vi "compare_command.vi"(11 "Command":string) -> (2 "Unknown":bool=TRUE, 3 "Count":i32=40)   [LabVIEW 2014]
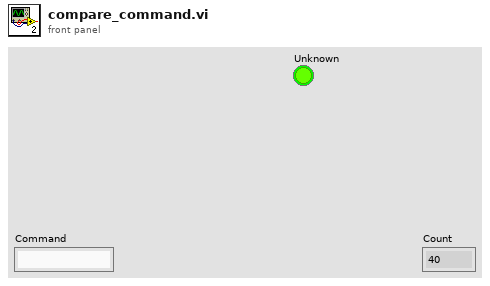
[diagram p1: front panel]
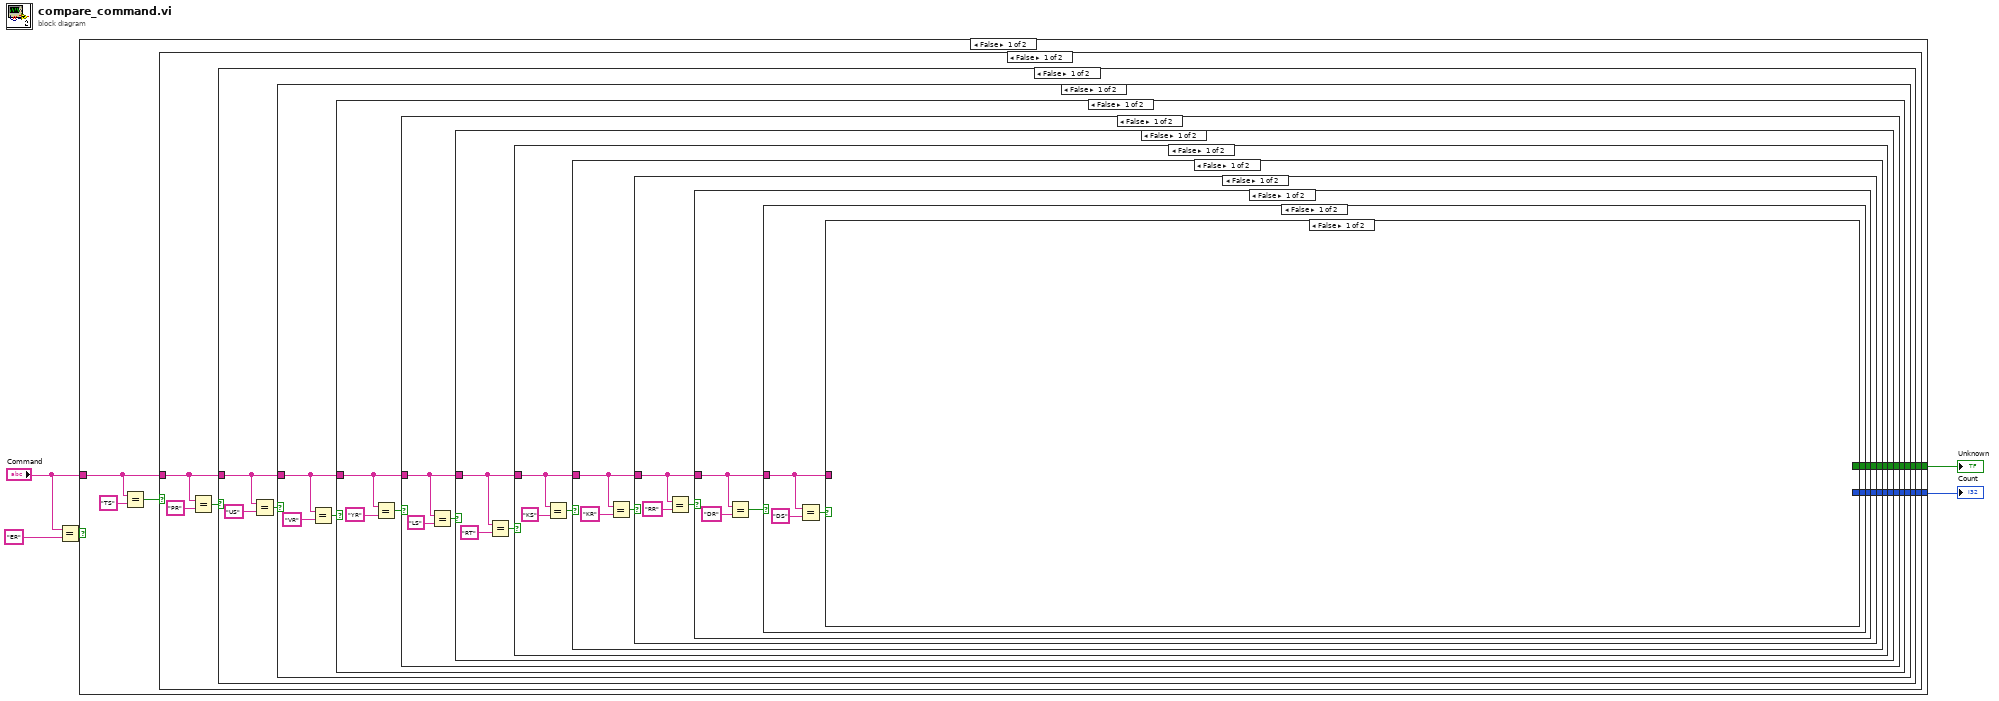
[diagram p0: block diagram]
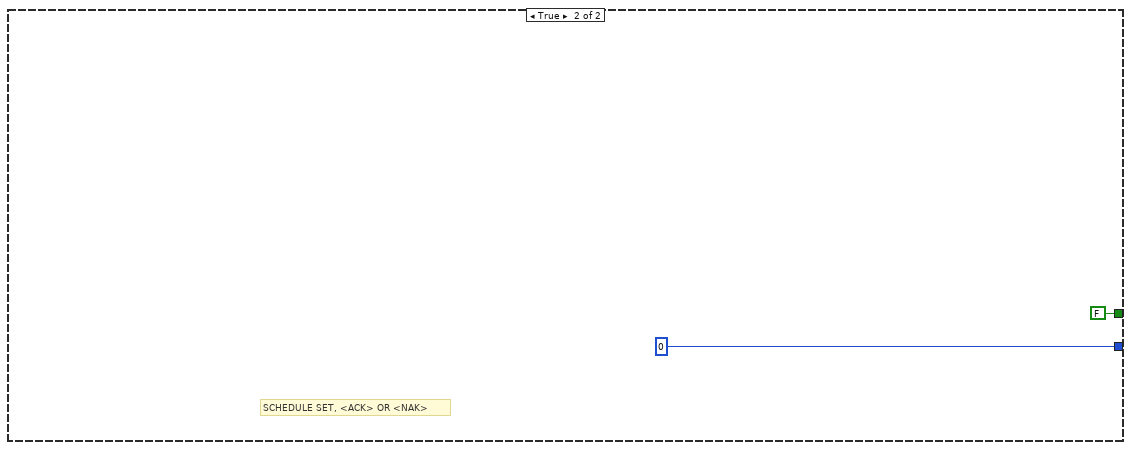
[diagram p2: hidden frame]
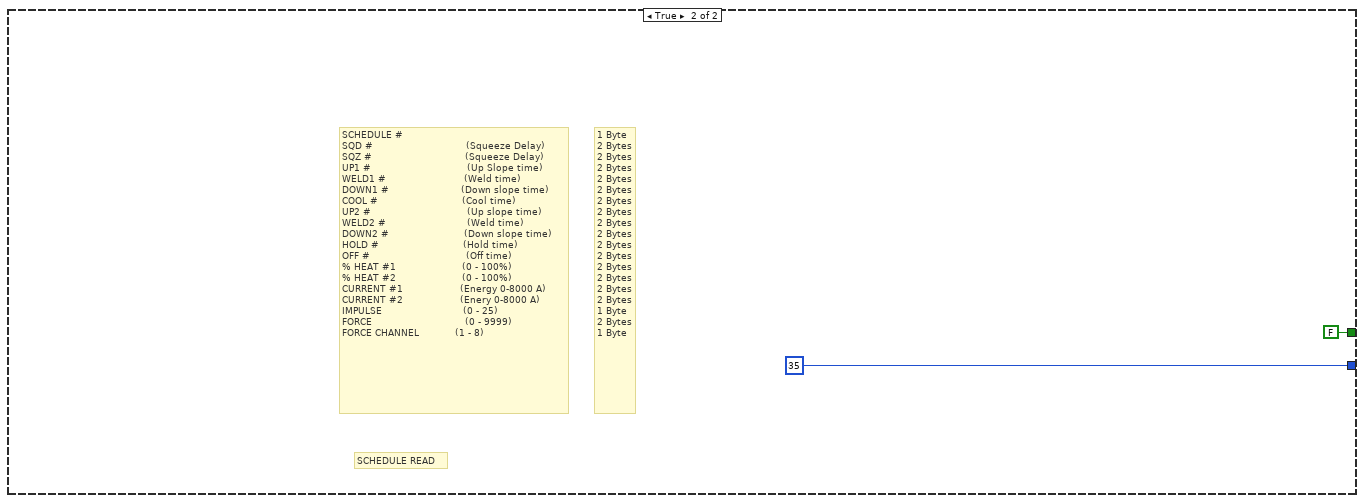
[diagram p3: hidden frame]
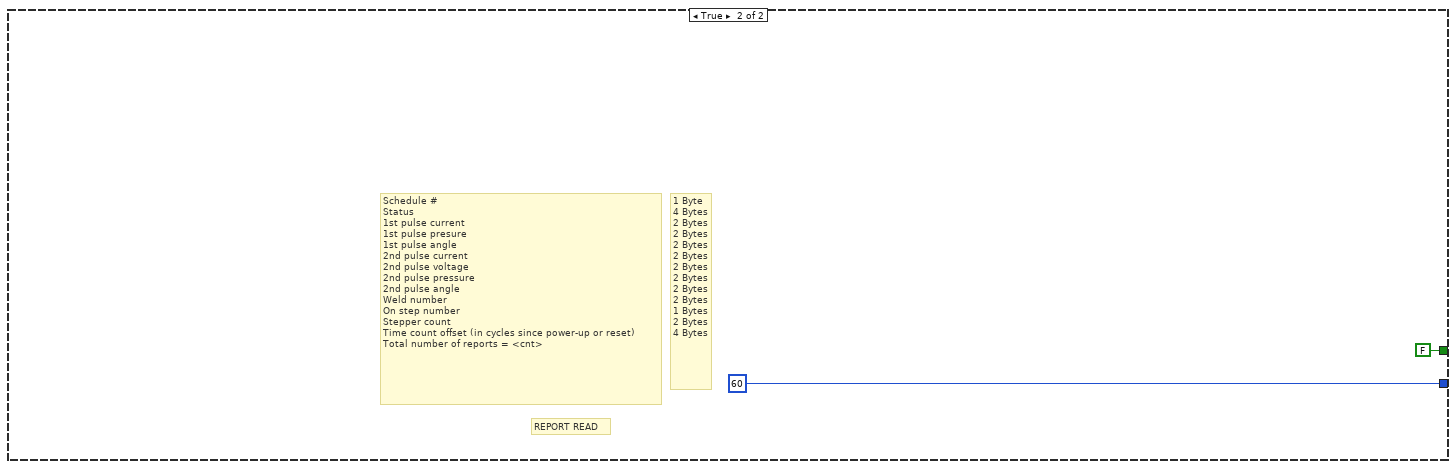
[diagram p4: hidden frame]
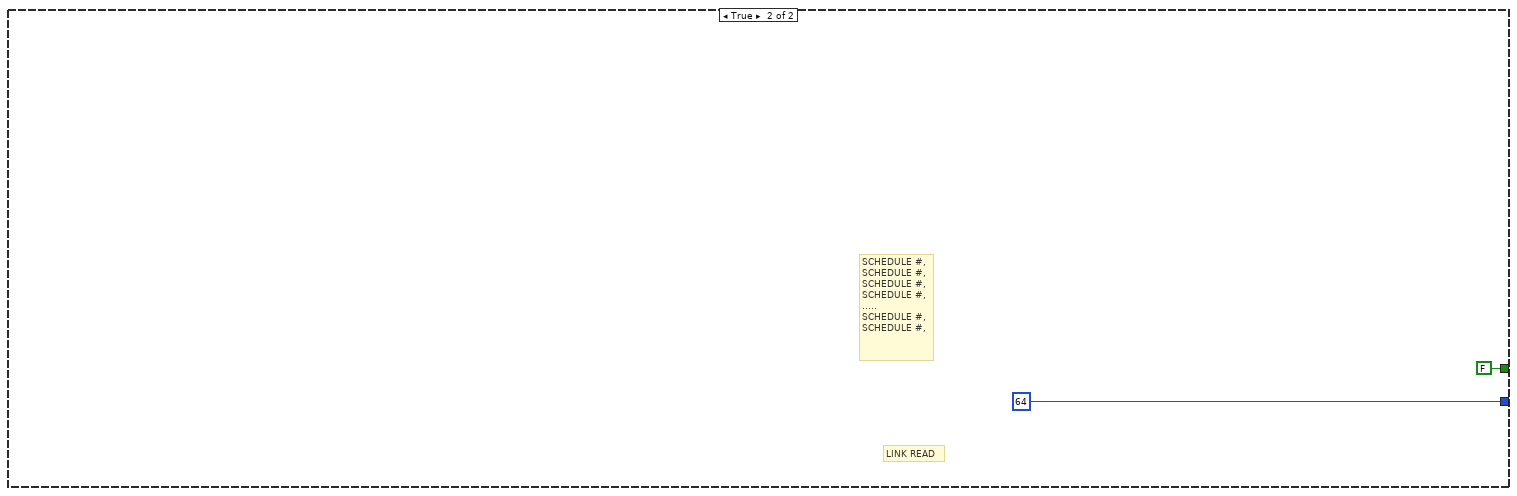
[diagram p5: hidden frame]
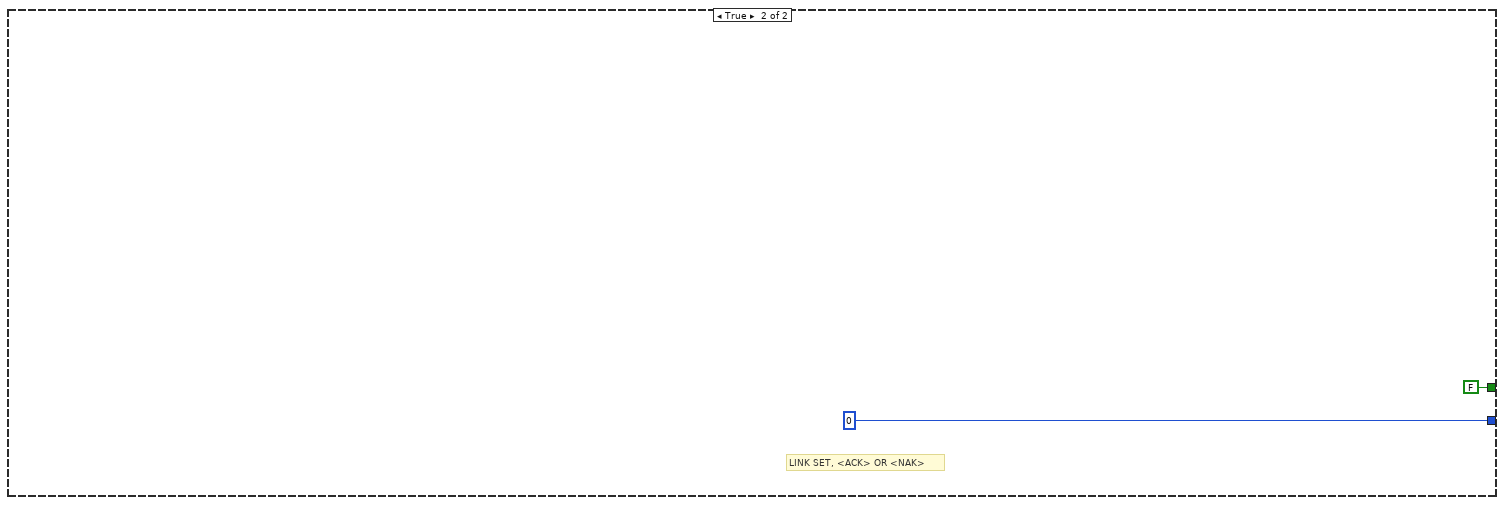
[diagram p6: hidden frame]
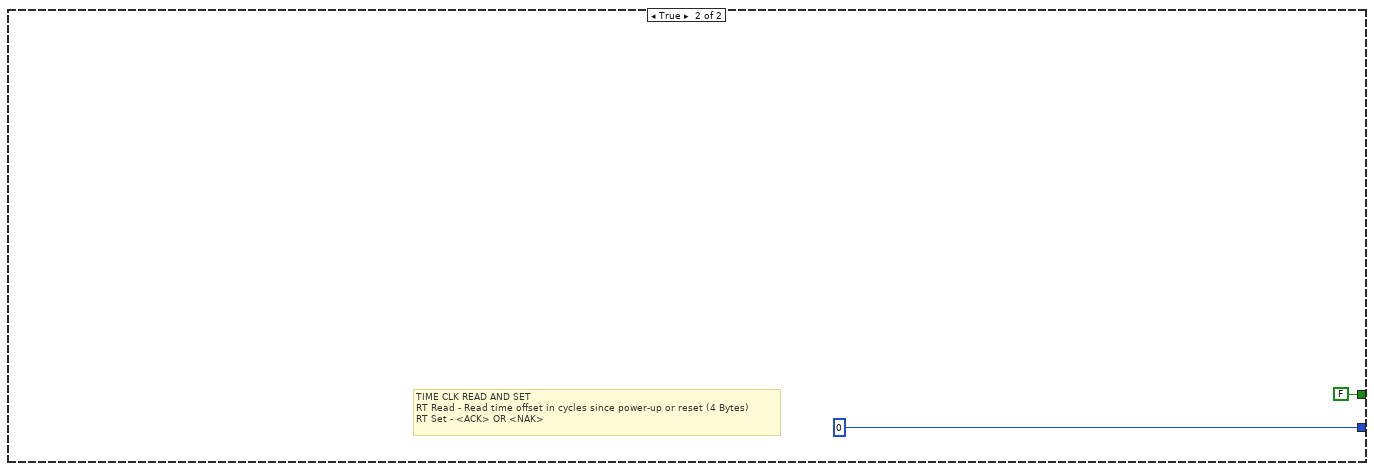
[diagram p7: hidden frame]
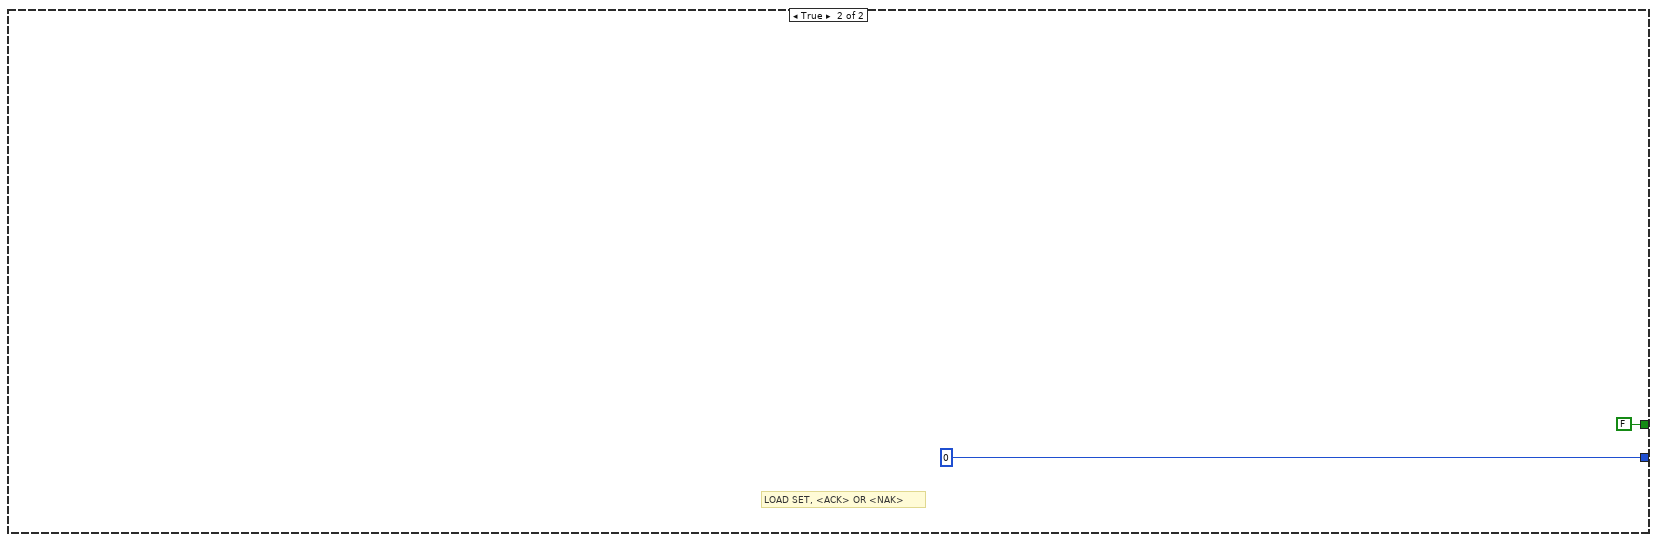
[diagram p8: hidden frame]
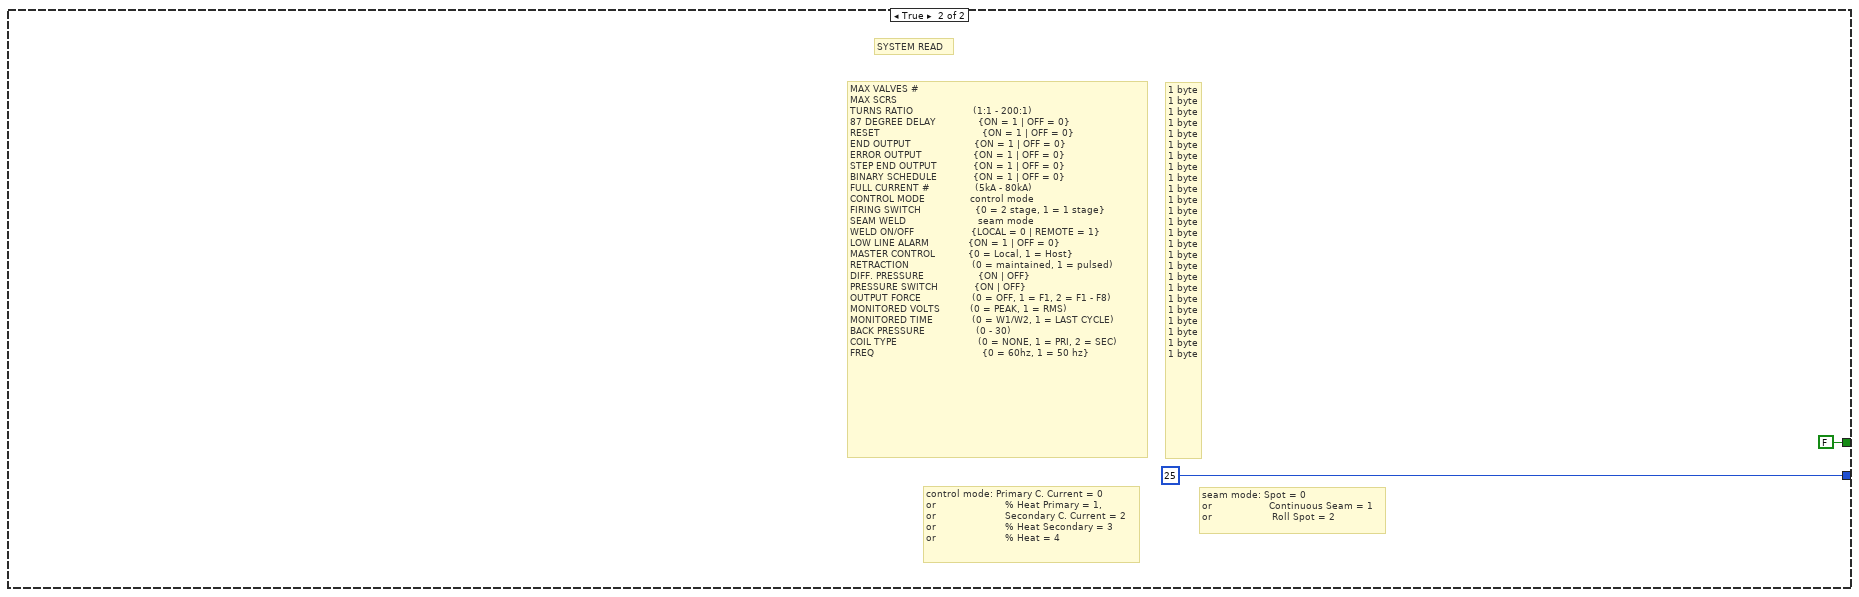
[diagram p9: hidden frame]
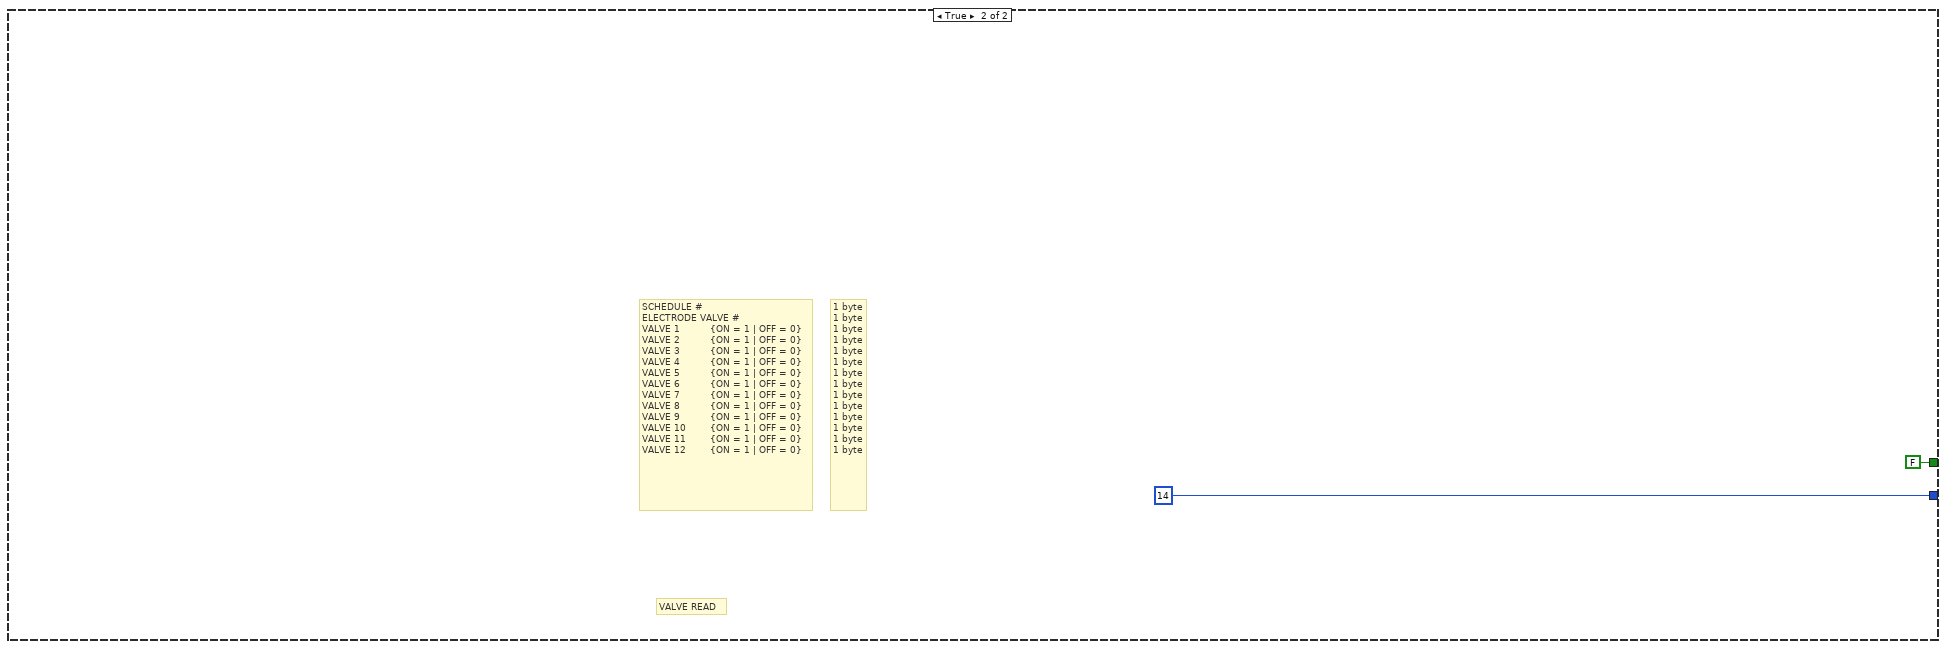
[diagram p10: hidden frame]
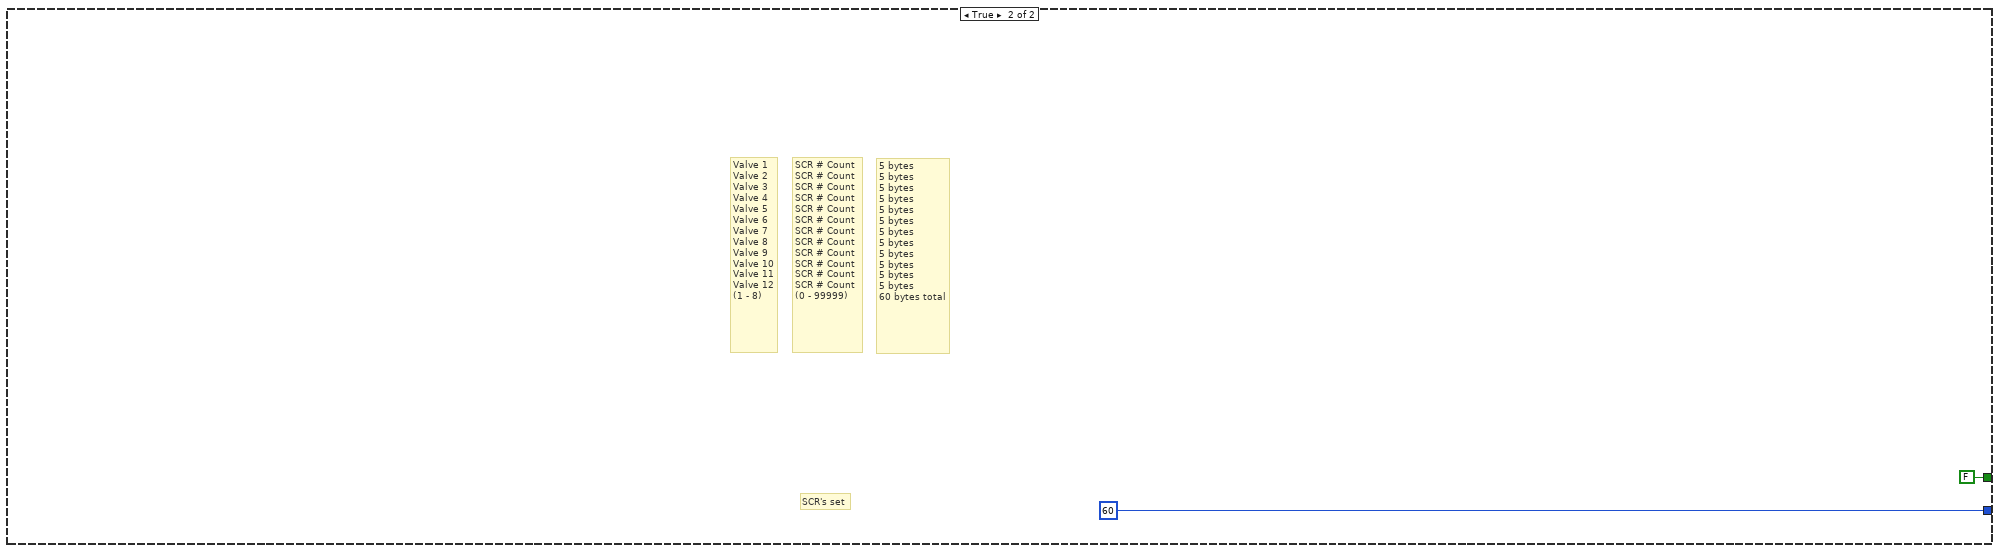
[diagram p11: hidden frame]
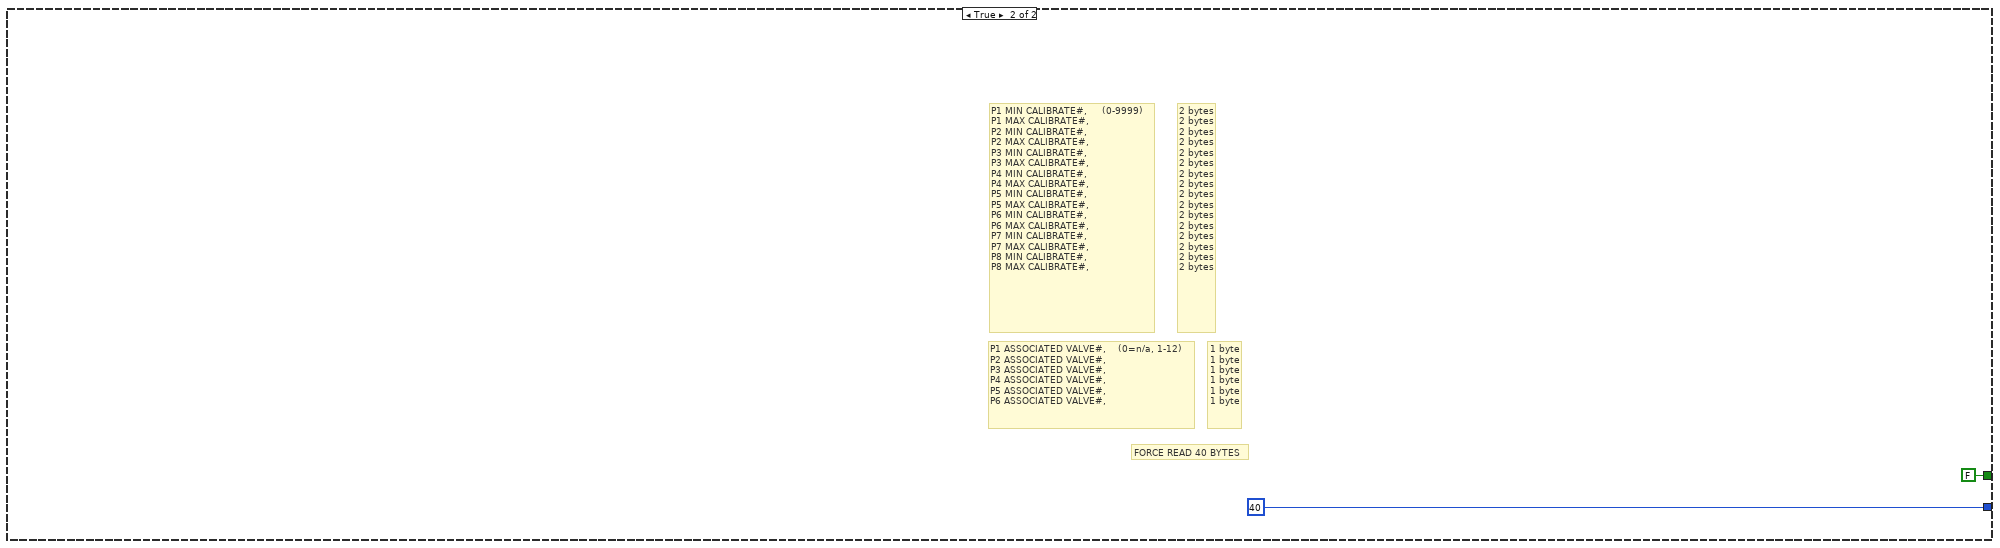
[diagram p12: hidden frame]
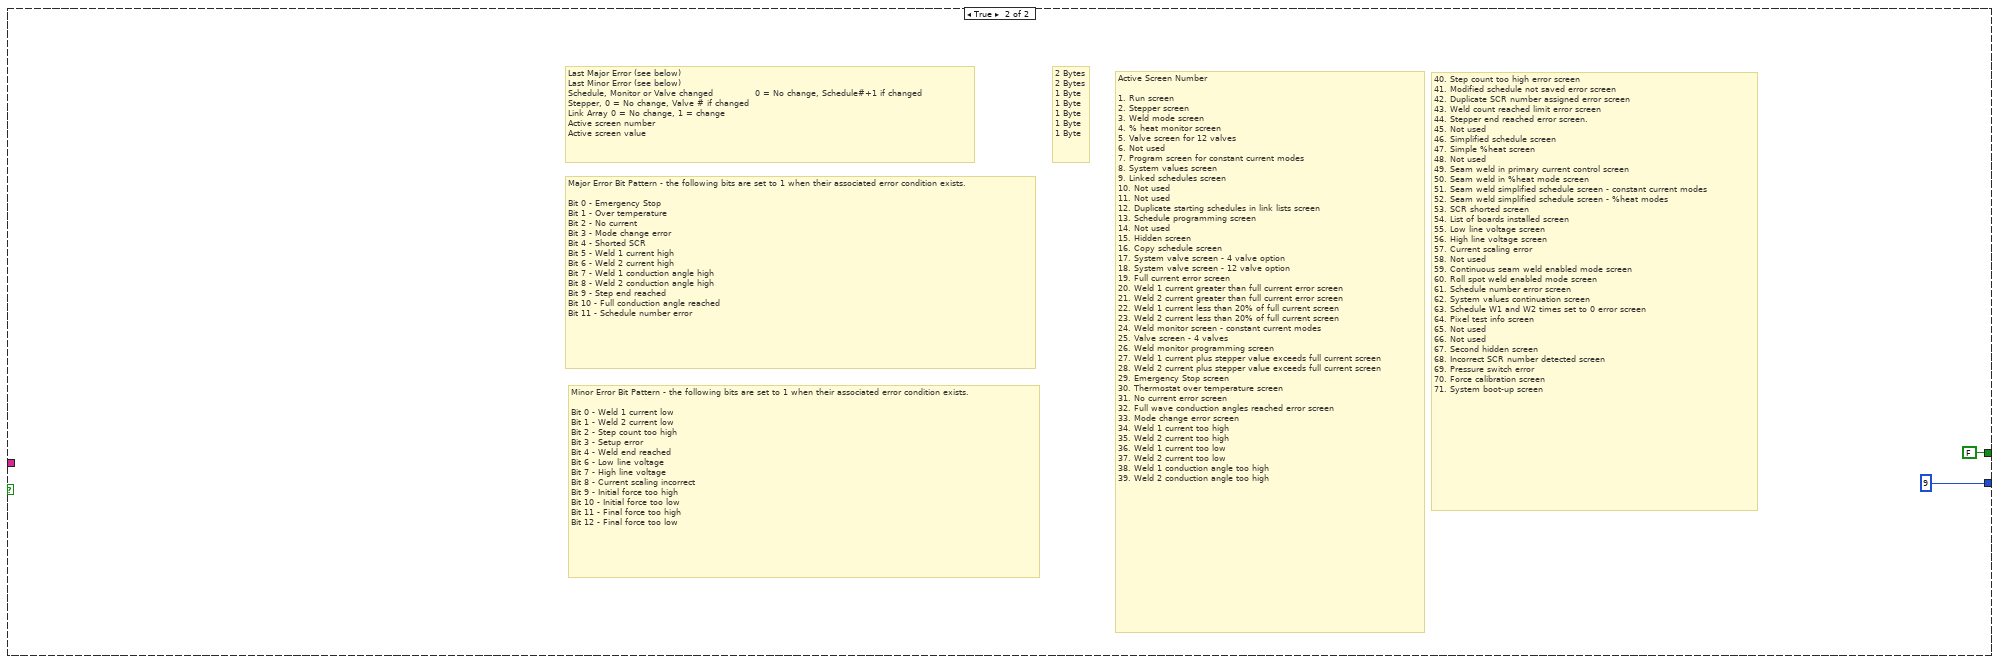
[diagram p13: hidden frame]
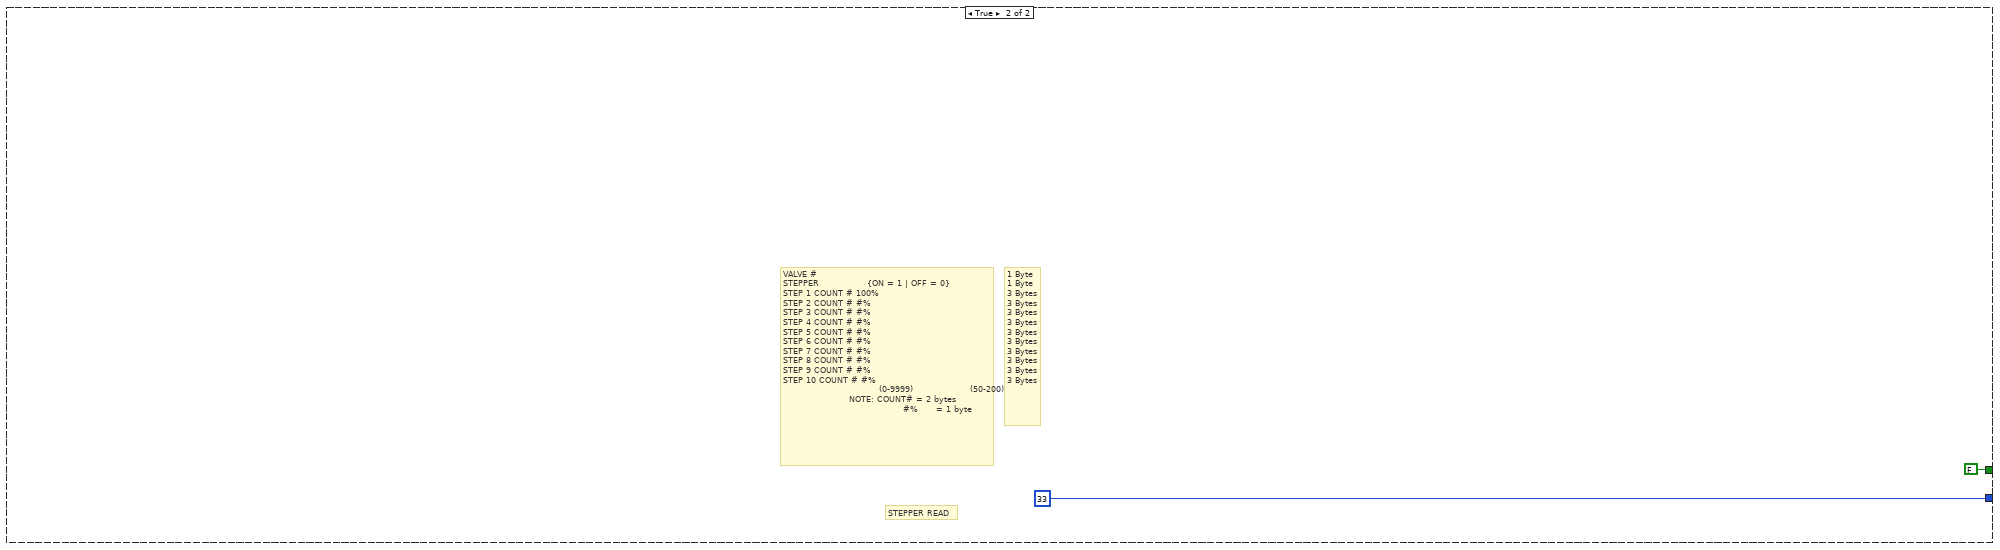
[diagram p14: hidden frame]
diagram:
  n1 = Equal?(x="Command", y="ER") -> (x = y?=w4:bool)
  n2 = case shown="False" w4 {
    tunnel: "Command" -> [w8 _]
    tunnel: [w10 33] -> w2
    tunnel: [w6 FALSE] -> w1
    frame False {
      n3 = Equal?(x=w8, y="TS") -> (x = y?=w7:bool)
      n4 = case shown="False" w7 {
        tunnel: w8 -> [w13 _]
        tunnel: [w12 9] -> w10
        tunnel: [w11 FALSE] -> w6
        frame False {
          n5 = Equal?(x=w13, y="PR") -> (x = y?=w14:bool)
          n6 = case shown="False" w14 {
            tunnel: w13 -> [w18 _]
            tunnel: [w17 40] -> w12
            tunnel: [w16 FALSE] -> w11
            frame False {
              n7 = Equal?(x=w18, y="US") -> (x = y?=w19:bool)
              n8 = case shown="False" w19 {
                tunnel: w18 -> [w22 _]
                tunnel: [w23 60] -> w17
                tunnel: [w21 FALSE] -> w16
                frame False {
                  n9 = Equal?(x=w22, y="VR") -> (x = y?=w24:bool)
                  n10 = case shown="False" w24 {
                    tunnel: w22 -> [w28 _]
                    tunnel: [w27 14] -> w23
                    tunnel: [w26 FALSE] -> w21
                    frame False {
                      n11 = Equal?(x=w28, y="YR") -> (x = y?=w29:bool)
                      n12 = case shown="False" w29 {
                        tunnel: w28 -> [w33 _]
                        tunnel: [w32 25] -> w27
                        tunnel: [w31 FALSE] -> w26
                        frame False {
                          n13 = Equal?(x=w33, y="LS") -> (x = y?=w34:bool)
                          n14 = case shown="False" w34 {
                            tunnel: w33 -> [w38 _]
                            tunnel: [w37 0] -> w32
                            tunnel: [w36 FALSE] -> w31
                            frame False {
                              n15 = Equal?(x=w38, y="RT") -> (x = y?=w39:bool)
                              n16 = case shown="False" w39 {
                                tunnel: w38 -> [w43 _]
                                tunnel: [w42 0] -> w37
                                tunnel: [w41 FALSE] -> w36
                                frame False {
                                n17 = Equal?(x=w43, y="KS") -> (x = y?=w44:bool)
                                n18 = case shown="False" w44 {
                                tunnel: w43 -> [w48 _]
                                tunnel: [w47 0] -> w42
                                tunnel: [w46 FALSE] -> w41
                                frame False {
                                n19 = Equal?(x=w48, y="KR") -> (x = y?=w49:bool)
                                n20 = case shown="False" w49 {
                                tunnel: w48 -> [w53 _]
                                tunnel: [w52 64] -> w47
                                tunnel: [w51 FALSE] -> w46
                                frame False {
                                n21 = Equal?(x=w53, y="RR") -> (x = y?=w54:bool)
                                n22 = case shown="False" w54 {
                                tunnel: w53 -> [w58 _]
                                tunnel: [w57 60] -> w52
                                tunnel: [w56 FALSE] -> w51
                                frame False {
                                n23 = Equal?(x=w58, y="DR") -> (x = y?=w59:bool)
                                n24 = case shown="False" w59 {
                                tunnel: w58 -> [w63 _]
                                tunnel: [w62 35] -> w57
                                tunnel: [w61 FALSE] -> w56
                                frame False {
                                n25 = Equal?(x=w63, y="DS") -> (x = y?=w64:bool)
                                n26 = case shown="False" w64 {
                                tunnel: w63 -> [w68 _]
                                tunnel: [w67 0] -> w62
                                tunnel: [w66 FALSE] -> w61
                                frame False {
                                n27 = Equal?(x=w68, y="MR") -> (x = y?=w69:bool)
                                n28 = case shown="False" w69 {
                                tunnel: w68 -> [w73 _]
                                tunnel: [w72 29] -> w67
                                tunnel: [w71 FALSE] -> w66
                                frame False {
                                n29 = Equal?(x=w73, y="MS") -> (x = y?=w74:bool)
                                n30 = case shown="False" w74 {
                                tunnel: w73 -> [w79 _]
                                tunnel: [w77 0] -> w72
                                tunnel: [w76 FALSE] -> w71
                                frame False {
                                n31 = Equal?(x=w79, y="LR") -> (x = y?=w78:bool)
                                n32 = case shown="False" w78 {
                                tunnel: w79 -> [w83 _]
                                tunnel: [w82 1] -> w77
                                tunnel: [w81 FALSE] -> w76
                                frame False {
                                n33 = Equal?(x=w83, y="ES") -> (x = y?=w84:bool)
                                n34 = case shown="False" w84 {
                                tunnel: w83 -> [w88 _]
                                tunnel: [w87 0] -> w82
                                tunnel: [w86 FALSE] -> w81
                                frame False {
                                n35 = Equal?(x=w88, y="VS") -> (x = y?=w89:bool)
                                n36 = case shown="False" w89 {
                                tunnel: w88 -> [w93 _]
                                tunnel: [w92 0] -> w87
                                tunnel: [w91 FALSE] -> w86
                                frame False {
                                n37 = Equal?(x=w93, y="CP") -> (x = y?=w94:bool)
                                n38 = case shown="False" w94 {
                                tunnel: w93 -> [w98 _]
                                tunnel: [w97 0] -> w92
                                tunnel: [w96 FALSE] -> w91
                                frame False {
                                n39 = Equal?(x=w98, y="UR") -> (x = y?=w99:bool)
                                n40 = case shown="False" w99 {
                                tunnel: w98 -> [w103 _]
                                tunnel: [w102 0] -> w97
                                tunnel: [w101 FALSE] -> w96
                                frame False {
                                n41 = Equal?(x=w103, y="CS") -> (x = y?=w104:bool)
                                n42 = case shown="False" w104 {
                                tunnel: w103 -> [w108 _]
                                tunnel: [w107 0] -> w102
                                tunnel: [w106 FALSE] -> w101
                                frame False {
                                n43 = Equal?(x=w108, y="YS") -> (x = y?=w109:bool)
                                n44 = case shown="False" w109 {
                                tunnel: w108 -> [w113 _]
                                tunnel: [w112 0] -> w107
                                tunnel: [w111 FALSE] -> w106
                                frame False {
                                n45 = Equal?(x=w113, y="TY") -> (x = y?=w114:bool)
                                n46 = case shown="False" w114 {
                                tunnel: w113 -> [w118 _]
                                tunnel: [w117 12] -> w112
                                tunnel: [w116 FALSE] -> w111
                                frame False {
                                n47 = Equal?(x=w118, y="PS") -> (x = y?=w119:bool)
                                n48 = case shown="False" w119 {
                                tunnel: w118 -> [w124 _]
                                tunnel: [w122 0] -> w117
                                tunnel: [w121 FALSE] -> w116
                                frame False {
                                n49 = Equal?(x=w124, y="CT") -> (x = y?=w123:bool)
                                n50 = case shown="False" w123 {
                                tunnel: [-1 1] -> w122
                                tunnel: [TRUE FALSE] -> w121
                                frame False {
                                # "NO SE INDENTIFICÓ EL\nCOMANDO, REGRESA -1"
                                }
                                frame True {
                                # "# REPORTS STORED"
                                # "COUNT READ"
                                }
                                }
                                }
                                frame True {
                                # "FORCE SET\n<ACK> OR <NAK>"
                                }
                                }
                                }
                                frame True {
                                # "1B\n1B\n1B\n1B\n1B\n1B\n1B\n1B\n1B\n1B\n1B\n1B"
                                # "S\nT\nA\n\n0-9\n0-9\n.\n0-9\n0-9\n\nA-Z\nA-Z"
                                # "\"STA\", RELEASE # AND REVISION #\nEXAMPLE: \"STA 01.21 AB\""
                                # "TYPE READ"
                                }
                                }
                                }
                                frame True {
                                # "SYSTEM SET\n<ACK> OR <NAK>"
                                }
                                }
                                }
                                frame True {
                                # "COUNTER SET, <ACK> OR <NAK>"
                                }
                                }
                                }
                                frame True {
                                # "SCR's read, <ACK> OR <NAK>"
                                }
                                }
                                }
                                frame True {
                                # "COPY SET, <ACK> OR <NAK>"
                                }
                                }
                                }
                                frame True {
                                # "VALVE SET, <ACK> OR <NAK>"
                                }
                                }
                                }
                                frame True {
                                # "STEPPER SET, <ACK> OR <NAK>"
                                }
                                }
                                }
                                frame True {
                                # "LOAD READ"
                                # "THE ACTIVE SCHEDULE #"
                                }
                                }
                                }
                                frame True {
                                # "MONITOR SET, <ACK> OR <NAK>"
                                }
                                }
                                }
                                frame True {
                                # "start value: MAINTAINED = 0\nor                PULSED = 1\nor                LATCHED = 2\nor                SEAM = 3"
                                # "weld mode: SPOT = 0\nor                  REPEAT = 1\nor                  SUCCESSIVE = 2\nor                  CHANGING = 3"
                                # "MONITOR READ"
                                # "1 Byte\n2 Bytes\n2 Bytes\n2 Bytes\n2 Bytes\n1 Byte\n1 Byte\n2 Bytes\n1 Byte\n1 Byte\n2 Bytes\n2 Bytes\n2 Bytes\n2 Bytes\n2 Bytes\n2 Bytes"
                                # "SCHEDULE #\nHIGH1C                 High current #1 %\nLOW1C                  High current #1 %\nHIGH2C                 High current #1 %\nLOW2C                  High current #1 %\nANGLE LIMIT        Conduction limit #1\nANGLE LIMIT        Conduction limit #2\nLIMIT                     Weld count limit\nSTART                   Start value\nMODE                    Weld mode\nLOP                        Low pressure limit            (0-9999)\nHIP                         High pressure limit\nVOLTHIW1            W1 High volt limit            (0.00-9.99)\nVOLTLOW1           W1 Low volt limit\nVOLTHIW2            W2 High volt limit\nVOLTLOW2           W2 Low volt limit"
                                }
                                }
                                }
                                frame True {
                                # "SCHEDULE SET, <ACK> OR <NAK>"
                                }
                                }
                                }
                                frame True {
                                # "SCHEDULE READ"
                                # "1 Byte\n2 Bytes\n2 Bytes\n2 Bytes\n2 Bytes\n2 Bytes\n2 Bytes\n2 Bytes\n2 Bytes\n2 Bytes\n2 Bytes\n2 Bytes\n2 Bytes\n2 Bytes\n2 Bytes\n2 Bytes\n1 Byte\n2 Bytes\n1 Byte"
                                # "SCHEDULE #\nSQD #                               (Squeeze Delay)\nSQZ #                               (Squeeze Delay)\nUP1 #                                (Up Slope time)\nWELD1 #                          (Weld time)\nDOWN1 #                        (Down slope time)\nCOOL #                            (Cool time)\nUP2 #                                (Up slope time)\nWELD2 #                           (Weld time)\nDOWN2 #                         (Down slope time)\nHOLD #                            (Hold time)\nOFF #                                (Off time)\n% HEAT #1                      (0 - 100%)\n% HEAT #2                      (0 - 100%)\nCURRENT #1                   (Energy 0-8000 A)\nCURRENT #2                   (Enery 0-8000 A)\nIMPULSE                           (0 - 25)\nFORCE                               (0 - 9999)\nFORCE CHANNEL            (1 - 8)"
                                }
                                }
                                }
                                frame True {
                                # "1 Byte\n4 Bytes\n2 Bytes\n2 Bytes\n2 Bytes\n2 Bytes\n2 Bytes\n2 Bytes\n2 Bytes\n2 Bytes\n1 Bytes\n2 Bytes\n4 Bytes"
                                # "Schedule #\nStatus\n1st pulse current\n1st pulse presure\n1st pulse angle\n2nd pulse current\n2nd pulse voltage\n2nd pulse pressure\n2nd pulse angle\nWeld number\nOn step number\nStepper count\nTime count offset (in cycles since power-up or reset)\nTotal number of reports = <cnt>"
                                # "REPORT READ"
                                }
                                }
                                }
                                frame True {
                                # "LINK READ"
                                # "SCHEDULE #,\nSCHEDULE #,\nSCHEDULE #,\nSCHEDULE #,\n.....\nSCHEDULE #,\nSCHEDULE #,"
                                }
                                }
                                }
                                frame True {
                                # "LINK SET, <ACK> OR <NAK>"
                                }
                                }
                                }
                                frame True {
                                # "TIME CLK READ AND SET\nRT Read - Read time offset in cycles since power-up or reset (4 Bytes)\nRT Set - <ACK> OR <NAK>"
                                }
                              }
                            }
                            frame True {
                              # "LOAD SET, <ACK> OR <NAK>"
                            }
                          }
                        }
                        frame True {
                          # "SYSTEM READ"
                          # "1 byte\n1 byte\n1 byte\n1 byte\n1 byte\n1 byte\n1 byte\n1 byte\n1 byte\n1 byte\n1 byte\n1 byte\n1 byte\n1 byte\n1 byte\n1 byte\n1 byte\n1 byte\n1 byte\n1 byte\n1 byte\n1 byte\n1 byte\n1 byte\n1 byte"
                          # "seam mode: Spot = 0\nor                   Continuous Seam = 1\nor                    Roll Spot = 2"
                          # "control mode: Primary C. Current = 0\nor                       % Heat Primary = 1,\nor                       Secondary C. Current = 2\nor                       % Heat Secondary = 3\nor                       % Heat = 4"
                          # "MAX VALVES #\nMAX SCRS\nTURNS RATIO                    (1:1 - 200:1)\n87 DEGREE DELAY              {ON = 1 | OFF = 0} \nRESET                                  {ON = 1 | OFF = 0}\nEND OUTPUT                     {ON = 1 | OFF = 0}\nERROR OUTPUT                 {ON = 1 | OFF = 0}\nSTEP END OUTPUT            {ON = 1 | OFF = 0}\nBINARY SCHEDULE            {ON = 1 | OFF = 0}\nFULL CURRENT #               (5kA - 80kA)\nCONTROL MODE               control mode\nFIRING SWITCH                  {0 = 2 stage, 1 = 1 stage}\nSEAM WELD                        seam mode\nWELD ON/OFF                   {LOCAL = 0 | REMOTE = 1}\nLOW LINE ALARM             {ON = 1 | OFF = 0}\nMASTER CONTROL           {0 = Local, 1 = Host}\nRETRACTION                     (0 = maintained, 1 = pulsed)\nDIFF. PRESSURE                  {ON | OFF}\nPRESSURE SWITCH            {ON | OFF}\nOUTPUT FORCE                 (0 = OFF, 1 = F1, 2 = F1 - F8)\nMONITORED VOLTS          (0 = PEAK, 1 = RMS)\nMONITORED TIME             (0 = W1/W2, 1 = LAST CYCLE)\nBACK PRESSURE                 (0 - 30)\nCOIL TYPE                           (0 = NONE, 1 = PRI, 2 = SEC)\nFREQ                                    {0 = 60hz, 1 = 50 hz}"
                        }
                      }
                    }
                    frame True {
                      # "VALVE READ"
                      # "1 byte\n1 byte\n1 byte\n1 byte\n1 byte\n1 byte\n1 byte\n1 byte\n1 byte\n1 byte\n1 byte\n1 byte\n1 byte\n1 byte"
                      # "SCHEDULE #\nELECTRODE VALVE #\nVALVE 1          {ON = 1 | OFF = 0}\nVALVE 2          {ON = 1 | OFF = 0}\nVALVE 3          {ON = 1 | OFF = 0}\nVALVE 4          {ON = 1 | OFF = 0}\nVALVE 5          {ON = 1 | OFF = 0}\nVALVE 6          {ON = 1 | OFF = 0}\nVALVE 7          {ON = 1 | OFF = 0}\nVALVE 8          {ON = 1 | OFF = 0}\nVALVE 9          {ON = 1 | OFF = 0}\nVALVE 10        {ON = 1 | OFF = 0}\nVALVE 11        {ON = 1 | OFF = 0}\nVALVE 12        {ON = 1 | OFF = 0}"
                    }
                  }
                }
                frame True {
                  # "5 bytes\n5 bytes\n5 bytes\n5 bytes\n5 bytes\n5 bytes\n5 bytes\n5 bytes\n5 bytes\n5 bytes\n5 bytes\n5 bytes\n60 bytes total"
                  # "SCR # Count\nSCR # Count\nSCR # Count\nSCR # Count\nSCR # Count\nSCR # Count\nSCR # Count\nSCR # Count\nSCR # Count\nSCR # Count\nSCR # Count\nSCR # Count\n(0 - 99999)"
                  # "Valve 1\nValve 2\nValve 3\nValve 4\nValve 5\nValve 6\nValve 7\nValve 8\nValve 9\nValve 10\nValve 11\nValve 12\n(1 - 8)"
                  # "SCR's set"
                }
              }
            }
            frame True {
              # "1 byte\n1 byte\n1 byte\n1 byte\n1 byte\n1 byte"
              # "2 bytes\n2 bytes\n2 bytes\n2 bytes\n2 bytes\n2 bytes\n2 bytes\n2 bytes\n2 bytes\n2 bytes\n2 bytes\n2 bytes\n2 bytes\n2 bytes\n2 bytes\n2 bytes"
              # "P1 ASSOCIATED VALVE#,    (0=n/a, 1-12)\nP2 ASSOCIATED VALVE#,\nP3 ASSOCIATED VALVE#,\nP4 ASSOCIATED VALVE#,\nP5 ASSOCIATED VALVE#,\nP6 ASSOCIATED VALVE#,"
              # "P1 MIN CALIBRATE#,     (0-9999)\nP1 MAX CALIBRATE#,\nP2 MIN CALIBRATE#,\nP2 MAX CALIBRATE#,\nP3 MIN CALIBRATE#,\nP3 MAX CALIBRATE#,\nP4 MIN CALIBRATE#,\nP4 MAX CALIBRATE#,\nP5 MIN CALIBRATE#,\nP5 MAX CALIBRATE#,\nP6 MIN CALIBRATE#,\nP6 MAX CALIBRATE#,\nP7 MIN CALIBRATE#,\nP7 MAX CALIBRATE#,\nP8 MIN CALIBRATE#,\nP8 MAX CALIBRATE#,"
              # "FORCE READ 40 BYTES"
            }
          }
        }
        frame True {
          # "40. Step count too high error screen\n41. Modified schedule not saved error screen\n42. Duplicate SCR number assigned error screen\n43. Weld count reached limit error screen\n44. Stepper end reached error screen.\n45. Not used\n46. Simplified schedule screen\n47. Simple %heat screen\n48. Not used\n49. Seam weld in primary current control screen\n50. Seam weld in %heat mode screen\n51. Seam weld simplified schedule screen - constant current modes\n52. Seam weld simplified schedule screen - %heat modes\n53. SCR shorted screen\n54. List of boards installed screen\n55. Low line voltage screen\n56. High line voltage screen\n57. Current scaling error\n58. Not used\n59. Continuous seam weld enabled mode screen\n60. Roll spot weld enabled mode screen\n61. Schedule number error screen\n62. System values continuation screen\n63. Schedule W1 and W2 times set to 0 error screen\n64. Pixel test info screen\n65. Not used\n66. Not used\n67. Second hidden screen\n68. Incorrect SCR number detected screen\n69. Pressure switch error\n70. Force calibration screen\n71. System boot-up screen"
          # "2 Bytes\n2 Bytes\n1 Byte\n1 Byte\n1 Byte\n1 Byte\n1 Byte"
          # "Active Screen Number\n\n1. Run screen\n2. Stepper screen\n3. Weld mode screen\n4. % heat monitor screen\n5. Valve screen for 12 valves\n6. Not used\n7. Program screen for constant current modes\n8. System values screen\n9. Linked schedules screen\n10. Not used\n11. Not used\n12. Duplicate starting schedules in link lists screen\n13. Schedule programming screen\n14. Not used\n15. Hidden screen\n16. Copy schedule screen\n17. System valve screen - 4 valve option\n18. System valve screen - 12 valve option\n19. Full current error screen\n20. Weld 1 current greater than full current error screen\n21. Weld 2 current greater than full current error screen\n22. Weld 1 current less than 20% of full current screen\n23. Weld 2 current less than 20% of full current screen\n24. Weld monitor screen - constant current modes\n25. Valve screen - 4 valves\n26. Weld monitor programming screen\n27. Weld 1 current plus stepper value exceeds full current screen\n28. Weld 2 current plus stepper value exceeds full current screen\n29. Emergency Stop screen\n30. Thermostat over temperature screen\n31. No current error screen\n32. Full wave conduction angles reached error screen\n33. Mode change error screen\n34. Weld 1 current too high\n35. Weld 2 current too high\n36. Weld 1 current too low\n37. Weld 2 current too low\n38. Weld 1 conduction angle too high\n39. Weld 2 conduction angle too high"
          # "Minor Error Bit Pattern - the following bits are set to 1 when their associated error condition exists.\n\nBit 0 - Weld 1 current low\nBit 1 - Weld 2 current low\nBit 2 - Step count too high\nBit 3 - Setup error\nBit 4 - Weld end reached\nBit 6 - Low line voltage\nBit 7 - High line voltage\nBit 8 - Current scaling incorrect\nBit 9 - Initial force too high\nBit 10 - Initial force too low\nBit 11 - Final force too high\nBit 12 - Final force too low"
          # "Major Error Bit Pattern - the following bits are set to 1 when their associated error condition exists.\n\nBit 0 - Emergency Stop\nBit 1 - Over temperature\nBit 2 - No current\nBit 3 - Mode change error\nBit 4 - Shorted SCR\nBit 5 - Weld 1 current high\nBit 6 - Weld 2 current high\nBit 7 - Weld 1 conduction angle high\nBit 8 - Weld 2 conduction angle high\nBit 9 - Step end reached\nBit 10 - Full conduction angle reached\nBit 11 - Schedule number error"
          # "Last Major Error (see below)\nLast Minor Error (see below)\nSchedule, Monitor or Valve changed              0 = No change, Schedule#+1 if changed\nStepper, 0 = No change, Valve # if changed\nLink Array 0 = No change, 1 = change\nActive screen number\nActive screen value"
        }
      }
    }
    frame True {
      # "STEPPER READ"
      # "1 Byte\n1 Byte\n3 Bytes\n3 Bytes\n3 Bytes\n3 Bytes\n3 Bytes\n3 Bytes\n3 Bytes\n3 Bytes\n3 Bytes\n3 Bytes"
      # "VALVE #\nSTEPPER                {ON = 1 | OFF = 0}\nSTEP 1 COUNT # 100%\nSTEP 2 COUNT # #%\nSTEP 3 COUNT # #%\nSTEP 4 COUNT # #%\nSTEP 5 COUNT # #%\nSTEP 6 COUNT # #%\nSTEP 7 COUNT # #%\nSTEP 8 COUNT # #%\nSTEP 9 COUNT # #%\nSTEP 10 COUNT # #%\n                                (0-9999)                   (50-200)\n                      NOTE: COUNT# = 2 bytes\n                                        #%      = 1 byte"
    }
  }
  "Count" <- w2
  "Unknown" <- w1
